vi "Set Bits U16.vi"(8 "Value (0)":u16 format="%b", 9 "Length (1)":u8=1, 10 "Start Index (0)":u8, 11 "Register in":u16 format="%032b") -> (1 "Length out":u8, 2 "Start Index out":u8, 3 "Register out":u16 format="%032b")   [LabVIEW 2016, in "GE 5565PIORC.lvclass"]
uses:
  GE 5565PIORC.lvclass
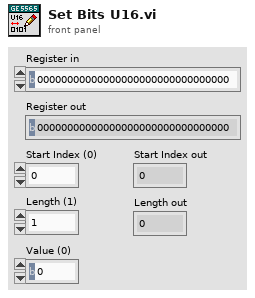
[diagram p1: front panel]
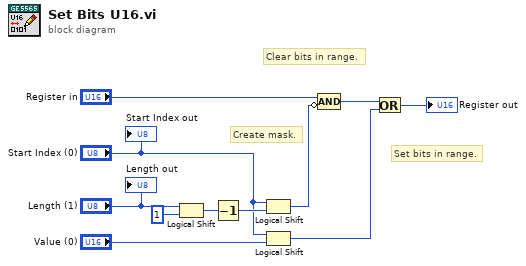
[diagram p0: block diagram]
diagram:
  # "Set bits in range."
  # "Create mask."
  # "Clear bits in range."
  n1 = Logical Shift(y="Length (1)", x=u16 1) -> (x << y=w4:u16)
  n2 = Decrement(x=w4) -> (x-1=w8:u16)
  n3 = Logical Shift(y="Start Index (0)", x=w8) -> (x << y=w1:u16)
  n4 = Logical Shift(y="Start Index (0)", x="Value (0)") -> (x << y=w2:u16)
  n5 = Compound Arithmetic op=AND("Register in", invert w1) -> (w9:u16)
  n6 = Or(x=w9, y=w2) -> (x .or. y?=→"Register out":u16)
  "Start Index out" <- "Start Index (0)"
  "Length out" <- "Length (1)"
